vi "Calculate Job Name and Path.vi"(9 "Job Target":string, 10 "Data in":variant, 11 "Build Job":refnum<class "Build Job.lvclass">) -> (0 "Workspace Path":string, 1 "Job Name":string, 2 "Data out":variant)   [LabVIEW 2014, in "Build Job.lvclass"]
uses:
  Build Job.lvclass
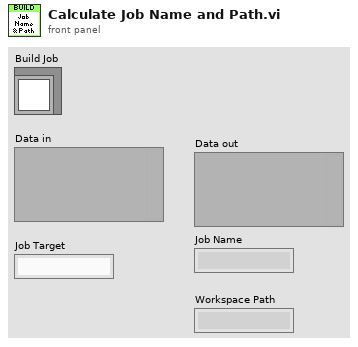
[diagram p1: front panel]
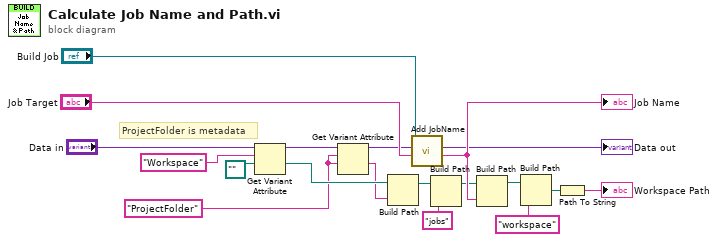
[diagram p0: block diagram]
diagram:
  w6 = "ProjectFolder"
  # "ProjectFolder is metadata"
  n1 = Get Variant Attribute(Variant="Data in", name="Workspace", default value (empty Variant)=path "") -> (duplicate Variant=w8:variant, value=w19:path)  [unwired: 1 in, 2 out]
  n2 = Get Variant Attribute(Variant=w8, name=w6, default value (empty Variant)=w6) -> (duplicate Variant=w3:variant, value=w1:string)  [unwired: 1 in, 2 out]
  n3 = Build Path(base path=w19, name or relative path=w1) -> (appended path=w15:path)
  n4 = call "Add JobName.vi"("Job Target"="Job Target", "Data in"=w3, "Build Job in"="Build Job") -> ("Job Name"=w18:string, "Data Out"=→"Data out":variant)  [unwired: 7 in]
  "Job Name" <- w18
  n5 = Build Path(base path=w15, name or relative path="jobs" ("string")) -> (appended path=w13:path)
  n6 = Build Path(base path=w13, name or relative path=w18) -> (appended path=w12:path)
  n7 = Build Path(base path=w12, name or relative path="workspace" ("string")) -> (appended path=w16:path)
  n8 = Path To String(path=w16) -> (string=→"Workspace Path":string)
